vi "PublishEnterOpStateTags.vi"(7 "op state":string, 8 "error in (no error)":errorcluster, 9 "data group name":string, 10 "operating states tags":variant, 11 "Qbus in":refnum<class "Qbus.lvclass">) -> (0 "error out":errorcluster)   [LabVIEW 2017, in "OpState.lvlib"]
uses:
  <vilib>/addons/InsightCM/Devices/Shared/Common/OpState/OpState.lvlib
  <vilib>/addons/Qbus/Qbus.lvclass
  <vilib>/addons/InsightCM/MessageBus/MessageLibrary/Tag/controls/TagUpdateStringValuesRoutedMessageBody.ctl
  <vilib>/addons/InsightCM/MessageBus/Base/controls/TagValueString.ctl
  <vilib>/addons/InsightCM/MessageBus/Base/controls/TsTagValueString.ctl
  <vilib>/addons/InsightCM/Devices/Shared/Common/ServerComm/ServerComm.lvlib
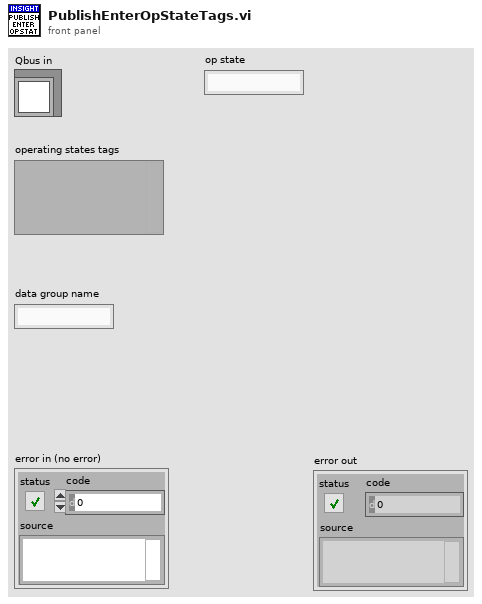
[diagram p1: front panel]
types:
  T1 = typedef "TagValueString.ctl" = cluster{"TagId":string, "TsValue":T2}
  T2 = typedef "TsTagValueString.ctl" = cluster{"Value":string, "Timestamp":i64}
  T3 = typedef "TagUpdateStringValuesRoutedMessageBody.ctl" = cluster{"TagsValue":T1[]}
  T4 = typedef "Message.ctl" = cluster{"Header":T5, "Body":u8[]}
  T5 = typedef "MessageHeader.ctl" = cluster{"MessageName":string, "Timestamp":i64, "CorrelationId":string, "ContentType":string, "RoutingKey":string, "Properties":T6[]}
  T6 = typedef "KeyValuePair.ctl" = cluster{"Key":string, "Value":string}
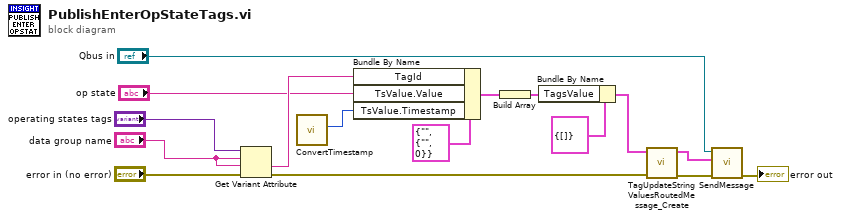
[diagram p0: block diagram]
diagram:
  n1 = Get Variant Attribute(Variant="operating states tags", name="data group name", default value (empty Variant)="data group name", error in="error in (no error)") -> (value=w3:string, error out=w1:errorcluster)  [unwired: 2 out]
  n2 = call <vilib>:"ConvertTimestamp.vi"() -> ("Timestamp out"=w5:i64)  [unwired: 11 in]
  n3 = Bundle By Name(cluster=T1 {"TagId"="", "TsValue"={"Value"="", "Timestamp"=0}} ("TagValue"), "TagId"=w3, "TsValue.Value"="op state", "TsValue.Timestamp"=w5) -> (w7:T1)
  n4 = Build Array(w7) -> (w9:T1[])
  n5 = Bundle By Name(cluster=T3 {"TagsValue"=[]} ("TagUpdateStringValuesRoutedMessage"), "TagsValue"=w9) -> (w6:T3)
  n6 = call <vilib>:"TagUpdateStringValuesRoutedMessage_Create.vi"("error in (no error)"=w1, "TagUpdateStringValuesRoutedMessage"=w6) -> ("error out"=w13:errorcluster, "Message"=w14:T4)  [unwired: 8 in]
  n7 = call <vilib>:"SendMessage.vi"("error in (no error)"=w13, "message"=w14, "Qbus in"="Qbus in") -> ("error out"=→"error out":errorcluster)  [unwired: 7 in, 1 out]
